vi "FGV_REWORK_DIAGNOSTICS_message_history_display.vi"(4 "front_panel_reference":refnum<vi>, 6 "SQL_listbox_reference":refnum<vi>, 7 "options":T1, 8 "error_in":errorcluster, 11 "input":variant) -> (0 "error_out":errorcluster)   [LabVIEW 2019]
uses:
  FGV_REWORK_DIAGNOSTICS_message_history_display.ctl
  FGV/DIAGNOSTICS_message_history_buffer/REWORK_DIAGNOSTICS_message_history_buffer_all_info.ctl
  _misc/DIAGNOSTICS_message_type.ctl
  _misc/AULocalize/SubVIs/Get Localized Phrase Compact Interface 1D.vi
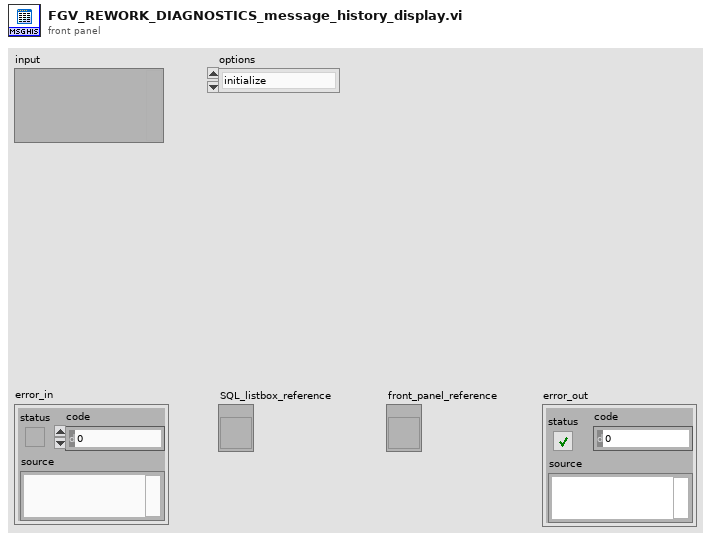
[diagram p1: front panel]
types:
  T1 = typedef "FGV_REWORK_DIAGNOSTICS_message_history_display.ctl" = enum16{"initialize", "display_messages"}
  T2 = typedef "REWORK_DIAGNOSTICS_message_history_buffer_all_info.ctl" = cluster{"timestamp":timestamp, "message_type":T3, "message":string, "record":string[]}
  T3 = typedef "DIAGNOSTICS_message_type.ctl" = enum16{"TCP", "SQL"}
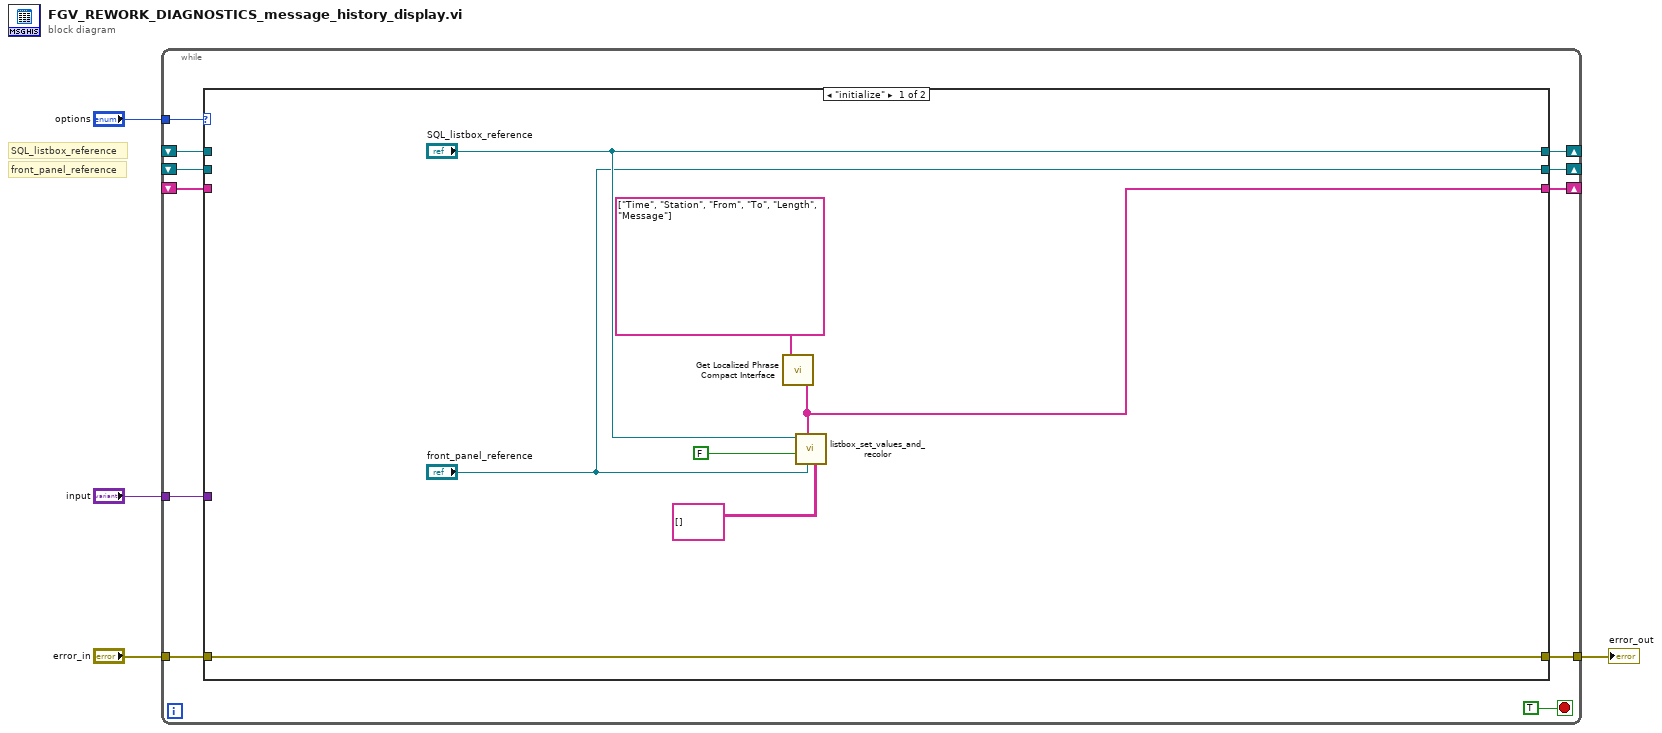
[diagram p0: block diagram]
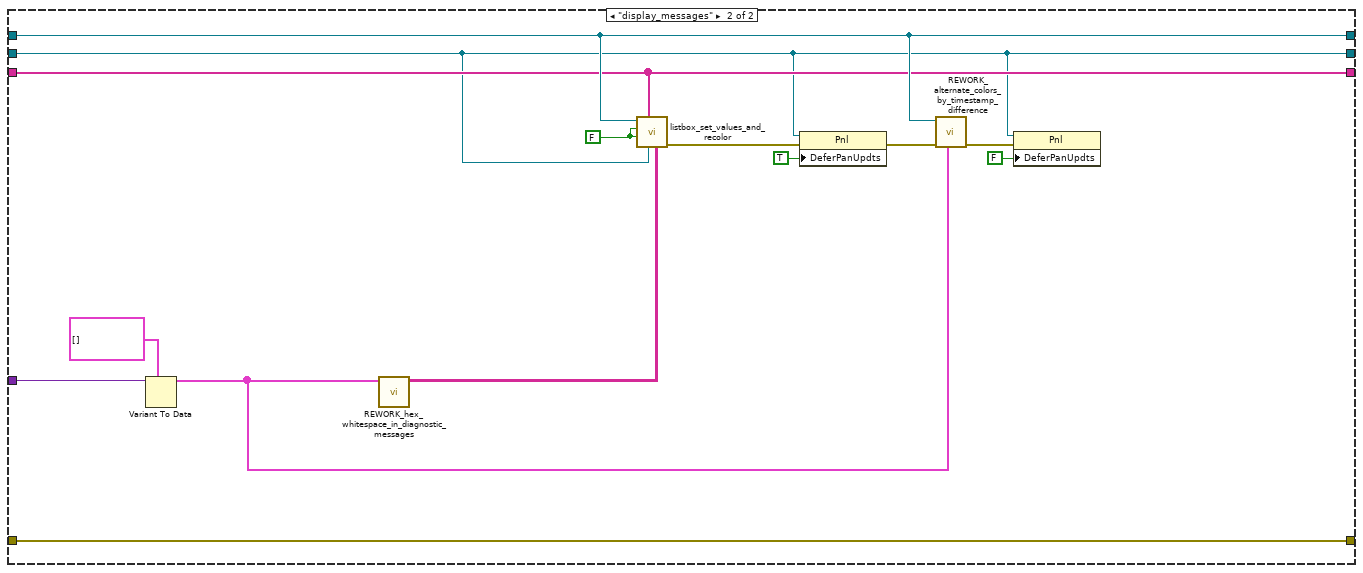
[diagram p2: hidden frame]
diagram:
  # "front_panel_reference"
  # "SQL_listbox_reference"
  n1 = while {
    tunnel: "options" -> [w14]
    tunnel: [w13] -> w4
    tunnel: "error_in" -> [w12]
    shift-right: [w11] -> _
    shift-left: _ -> [w10]
    tunnel: "input" -> [w9]
    shift-right: [w8] -> _
    shift-left: _ -> [w7]
    shift-right: [w6] -> _
    shift-left: _ -> [w5]
    stop <- TRUE stop-if-true
    n2 = case shown="\"initialize\"" w14 {
      tunnel: [w22 w36] -> w13
      tunnel: w12 -> [w22 w36]
      tunnel: ["SQL_listbox_reference" w30] -> w11
      tunnel: w10 -> [_ w30]
      tunnel: w9 -> [_ w35]
      tunnel: ["front_panel_reference" w25] -> w8
      tunnel: w7 -> [_ w25]
      tunnel: [w16 w27] -> w6
      tunnel: w5 -> [_ w27]
      frame "initialize" {
        n3 = call-poly "Get Localized Phrase Compact Interface.vi"("Key"=string[] ["Time", "Station", "From", "To", "Length", "Message"] ("column_names")) -> ("Translated Phrase"=w16:string[])
        n4 = call "listbox_set_values_and_recolor.vi"("item_names"=string[][] [], "front_panel_reference"="front_panel_reference", "column_names"=w16, "Autosize? (T)"=FALSE, "multicolumn_listbox_reference_in"="SQL_listbox_reference") -> ()  [unwired: 5 in, 2 out]
      }
      frame "display_messages" {
        w29 = FALSE ("Autosize? (T)")
        n5 = Variant To Data(type=T2[] [] ("message_history"), Variant=w35) -> (data=w31:T2[])  [unwired: 1 in, 1 out]
        n6 = call "REWORK_hex_whitespace_in_diagnostic_messages.vi"("message_history"=w31) -> ("hexed_records"=w28:string[][])  [unwired: 10 in]
        n7 = call "listbox_set_values_and_recolor.vi"("item_names"=w28, "front_panel_reference"=w25, "column_names"=w27, "Autosize? (T)"=w29, "Recolor? (T)"=w29, "multicolumn_listbox_reference_in"=w30) -> ("error_out"=w24:errorcluster)  [unwired: 4 in, 1 out]
        n8 = property on="Property Node" class="Pnl"(reference=w25, error in=w24, "DeferPanUpdts"=TRUE ("Defer Panel Updates")) -> (error out=w23:errorcluster)  [unwired: 1 out]
        n9 = call "REWORK_alternate_colors_by_timestamp_difference.vi"("message_history_buffer"=w31, "error_in"=w23, "listbox_ref"=w30) -> ("error_out"=w32:errorcluster)  [unwired: 8 in]
        n10 = property on="Property Node" class="Pnl"(reference=w25, error in=w32, "DeferPanUpdts"=FALSE ("Defer Panel Updates")) -> ()  [unwired: 2 out]
      }
    }
  }
  "error_out" <- w4
